vi "CloseSensorSession.vi"(8 "error in (no error)":errorcluster, 11 "RoomAlert in":refnum<class "RoomAlert.lvclass">) -> (0 "error out":errorcluster, 3 "RoomAlert out":refnum<class "RoomAlert.lvclass">)   [LabVIEW 2018, in "SensorPlugins.lvlib" / "RoomAlert.lvclass"]
uses:
  RoomAlert.lvclass
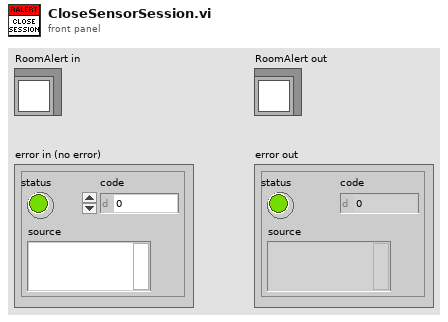
[diagram p1: front panel]
types:
  T1 = typedef "SensorPlugins.lvlib/RoomAlert.lvclass/RoomAlertControls.ctl" = cluster{"Connected?":bool, "IP Address of SNMP Device":string, "Port (502)":u16, "GET OID ARRAY":string[], "SET OID ARRAY":string[][], "Community Name":string, "OID":string[], "Measurements To Read Array":u16[], "Use Measurement To Read Array":bool}[]
  T2 = typedef "SensorPlugins.lvlib/RoomAlert.lvclass/CommunicationControls.ctl" = refnum<k16>[]
  T3 = cluster{"Connected?":bool, "IP Address of SNMP Device":string, "Port (502)":u16, "GET OID ARRAY":string[], "SET OID ARRAY":string[][], "Community Name":string, "OID":string[], "Measurements To Read Array":u16[], "Use Measurement To Read Array":bool}
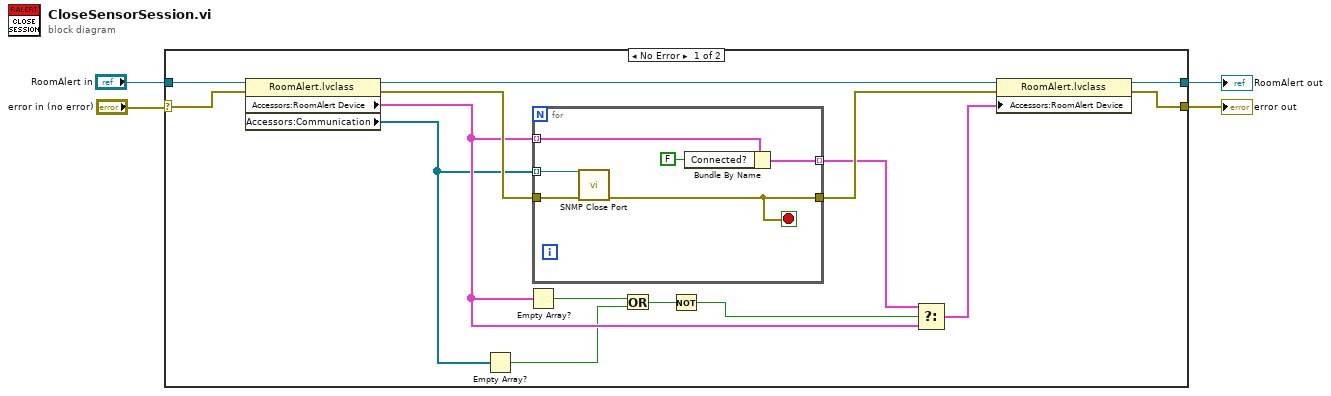
[diagram p0: block diagram]
diagram:
  n1 = case shown="No Error" "error in (no error)" {
    selector: "error in (no error)" -> [w18 w26]
    tunnel: "RoomAlert in" -> [w19 w27]
    tunnel: [w15 w27] -> w2
    tunnel: [w14 w26] -> w1
    frame No Error {
      n2 = property class="RoomAlert.lvclass"(reference=w19, error in=w18) -> (reference out=w16:refnum<class "RoomAlert.lvclass">, error out=w17:errorcluster, "Accessors:RoomAlert Device"=w10:T1, "Accessors:Communication "=w9:T2)
      n3 = Empty Array?(array=w9) -> (empty?=w7:bool)
      n4 = Empty Array?(array=w10) -> (empty?=w8:bool)
      n5 = for {
        tunnel: w17 -> [w22]
        tunnel: [w21] -> w13
        tunnel: w9 -> [w20] mode=indexing
        tunnel: w10 -> [w25] mode=indexing
        tunnel: [w23] -> w11 mode=indexing
        stop <- w21 stop-if-true
        n6 = call "SNMP Close Port.vi"("error in (no error)"=w22, "connection ID"=w20) -> ("error out"=w21:errorcluster)  [unwired: 9 out]
        n7 = Bundle By Name(cluster=w25, "Connected?"=FALSE) -> (w23:T3)
      }
      n8 = Or(x=w8, y=w7) -> (x .or. y?=w6:bool)
      n9 = Not(x=w6) -> (.not. x?=w12:bool)
      n10 = Select(t=w11, s=w12, f=w10) -> (s? t:f=w5:T1)
      n11 = property class="RoomAlert.lvclass"(reference=w16, error in=w13, "Accessors:RoomAlert Device"=w5) -> (reference out=w15:refnum<class "RoomAlert.lvclass">, error out=w14:errorcluster)
    }
    frame Error {
    }
  }
  "error out" <- w1
  "RoomAlert out" <- w2
